vi "TCP_GV.vi"() -> ()   [LabVIEW 2016]
panel:
  out "TCP Output":string
  in  "Bytes":dbl
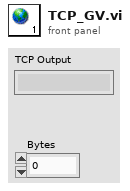
[diagram p1: front panel]
diagram:
